vi "Cluster to Array of Variants.vi"(10 "Cluster":variant) -> (2 "Array of Cluster Elements":variant[](array[variant]))   [LabVIEW 2024, in "JDP Utility.lvlib"]
doc: "Converts a Cluster into an Array of Variants containing the Cluster's elements."
uses:
  JDP Utility.lvlib
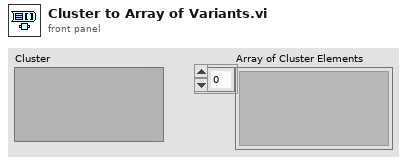
[diagram p1: front panel]
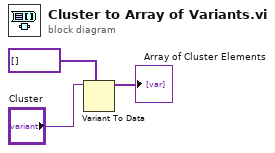
[diagram p0: block diagram]
diagram:
  n1 = Variant To Data(type=variant[] [] ("Array"), Variant="Cluster") -> (data=→"Array of Cluster Elements":variant[])  [unwired: 1 in, 1 out]
